vi "DestroyAllSessions.vi"(8 "error in (no error)":errorcluster) -> (0 "error out":errorcluster)   [LabVIEW 2017, in "libonnx_wrapper.lvlib"]
doc: "/**\n * @brief Уничтожить ВСЕ активные сессии (полная очистка памяти)\n * \n * Эта функция находит все созданные сессии в хранилище, освобождает их память,\n * удаляет метаданные и очищает список сессий. Полезно вызывать при завершении\n * работы приложения для гарантированного освобождения ресурсов.\n * \n * @return void\n * \n * @note После вызова все ранее полученные SessionID становятся невалидными\n * @note Не нужно вызывать DestroySession для каждой сессии отдельно\n * @note Безопасно вызывать, даже если сессий не было создано (ничего не сделает)\n */\nvoid DestroyAllSessions(void);"
uses:
  libonnx_wrapper.lvlib
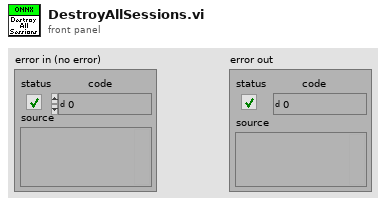
[diagram p1: front panel]
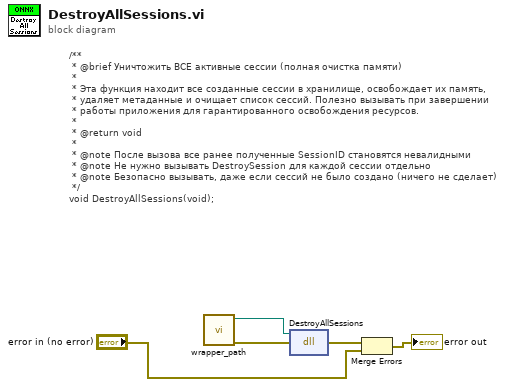
[diagram p0: block diagram]
diagram:
  # "/**\n * @brief Уничтожить ВСЕ активные сессии (полная очистка памяти)\n * \n * Эта функция находит все созданные сессии в хранилище, освобождает их память,\n * удаляет метаданные и очищает список сессий. Полезно вызывать при завершении\n * работы приложения для гарантированного освобождения ресурсов.\n * \n * @return void\n * \n * @note После вызова все ранее полученные SessionID становятся невалидными\n * @note Не нужно вызывать DestroySession для каждой сессии отдельно\n * @note Безопасно вызывать, даже если сессий не было создано (ничего не сделает)\n */\nvoid DestroyAllSessions(void);"
  n1 = call "wrapper_path.vi"() -> ("error out"=w4:errorcluster, "wrapper path"=w3:path)  [unwired: 10 in]
  n2 = dll-call lib="home/ivan/LabVIEWData/ONNX/Test/libonnx_wrapper/unix64/libonnx_wrapper.so" fn="DestroyAllSessions"(path in=w3, error in=w4) -> (error out=w5:errorcluster)  [unwired: 2 in, 1 out]
  n3 = Merge Errors(w5, "error in (no error)") -> (→"error out":errorcluster)
